vi "canencode.vi"(10 "lock":bool) -> (2 "CAN Write":T1={"timestamp high"=0, "timestamp low"=0, "identifier"=0, "type"=enum."Data Frame", "info A"=0, "info B"=0, "data length"=0, "data"=[0, 0, 0, 0, 0, 0, 0, 0]})   [LabVIEW 2012]
uses:
  RIOGlobal.vi
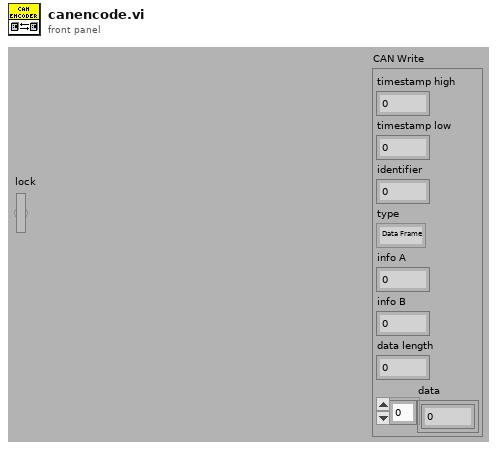
[diagram p1: front panel]
types:
  T1 = cluster{"timestamp high":u32, "timestamp low":u32, "identifier":u32, "type":enum8{"Data Frame", "Remote Frame", "(reserved)", "(reserved) ", "(reserved)  ", "(reserved)   ", "Bus Error", "Transceiver Fault"}, "info A":u8, "info B":u8, "data length":u8, "data":u8[]}
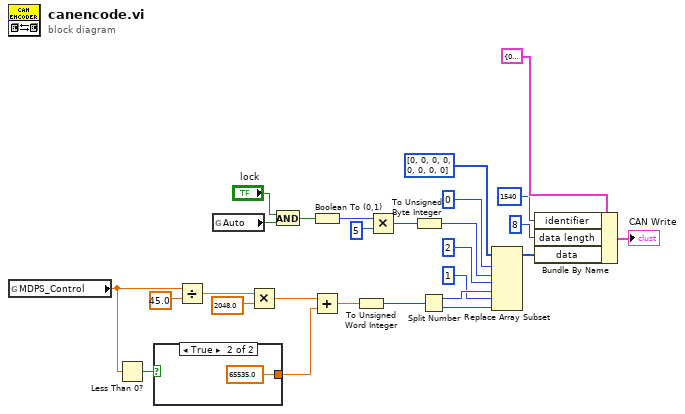
[diagram p0: block diagram]
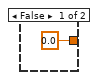
[diagram p2: hidden frame]
diagram:
  n1 = global read "RIOGlobal.vi" "MDPS_Control"() -> (w1:dbl)
  n2 = Less Than 0?(x=w1) -> (x < 0?=w21:bool)
  n3 = case shown="True" w21 {
    tunnel: [0.0 ("y") 65535.0 ("y")] -> w19
    frame False {
    }
    frame True {
    }
  }
  n4 = Divide(x=w1, y=45.0) -> (x/y=w23:dbl)
  n5 = global read "RIOGlobal.vi" "Auto"() -> (w2:bool)
  n6 = Multiply(x=w23, y=2048.0) -> (x*y=w20:dbl)
  n7 = And(x="lock", y=w2) -> (x .and. y?=w15:bool)
  n8 = Boolean To (0,1)(Boolean=w15) -> (0, 1=w27:i16)
  n9 = Add(x=w20, y=w19) -> (x+y=w18:dbl)
  n10 = To Unsigned Word Integer(number=w18) -> (unsigned 16bit integer=w17:u16)
  n11 = Multiply(x=w27, y=i16 5) -> (x*y=w25:i16)
  n12 = To Unsigned Byte Integer(number=w25) -> (unsigned 8bit integer=w10:u8)
  n13 = Split Number(x=w17) -> (hi(x)=w7:u8, lo(x)=w5:u8)
  n14 = Replace Array Subset(array=u8[] [0, 0, 0, 0, 0, 0, 0, 0] ("data"), new element #1=w10, index #1=0 ("index"), new element #2=w7, index #2=2 ("index"), new element #3=w5, index #3=1 ("index")) -> (w3:u8[])
  n15 = Bundle By Name(cluster=T1 {"timestamp high"=0, "timestamp low"=0, "identifier"=0, "type"=enum."Data Frame", "info A"=0, "info B"=0, "data length"=0, "data"=[0, 0, 0, 0, 0, 0, 0, 0]} ("CAN Write"), "identifier"=u32 1540, "data length"=u8 8, "data"=w3) -> (→"CAN Write":T1)
